vi "RS_RF_commands.vi"(1 "Value":dbl, 2 "Parameter":T1(ring)) -> (0 "Command":string)   [LabVIEW 2013]
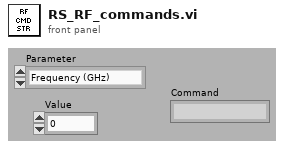
[diagram p1: front panel]
types:
  T1 = enum16{"Frequency (GHz)", "Power (dBm)", "Pulse period (us)", "Pulse width (us)", "Pulse delay (us)", "Pulse modulation?", "Output on?", "Pulse source", "Pulse mode", "Trigger mode", "Ex trigger input slope", "External impedance"}
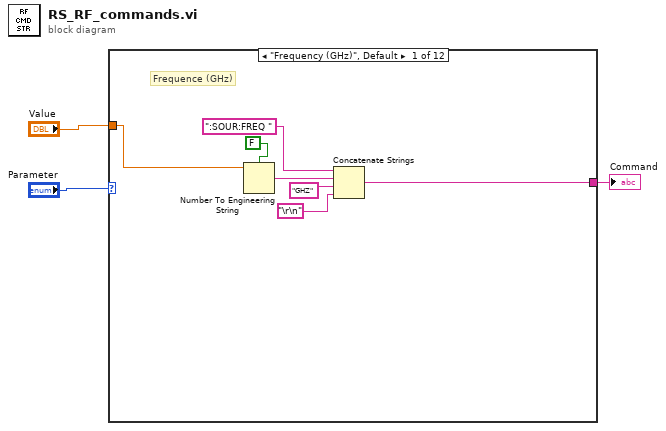
[diagram p0: block diagram]
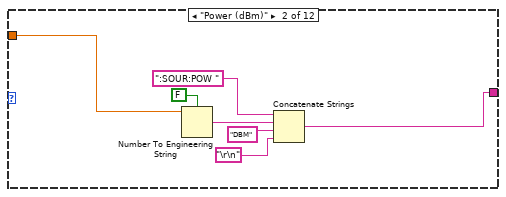
[diagram p2: hidden frame]
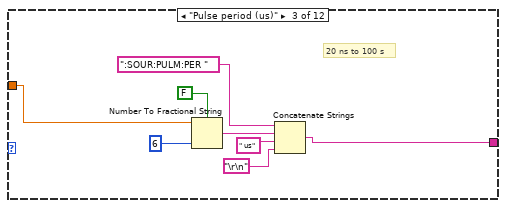
[diagram p3: hidden frame]
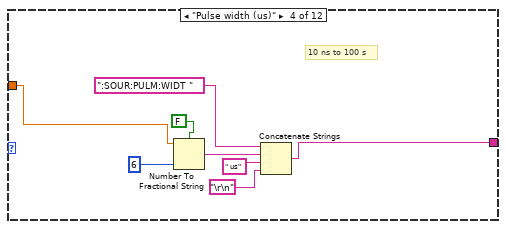
[diagram p4: hidden frame]
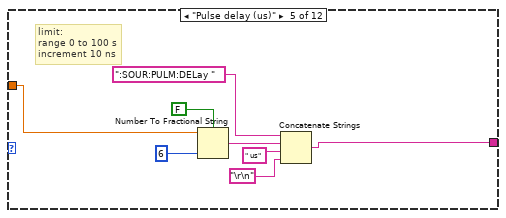
[diagram p5: hidden frame]
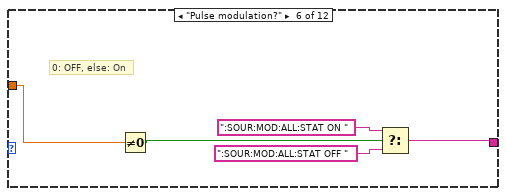
[diagram p6: hidden frame]
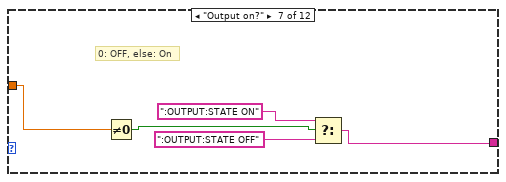
[diagram p7: hidden frame]
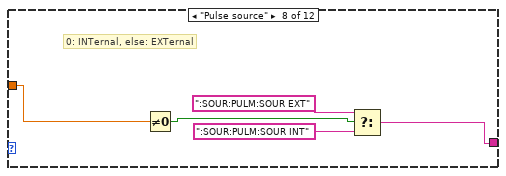
[diagram p8: hidden frame]
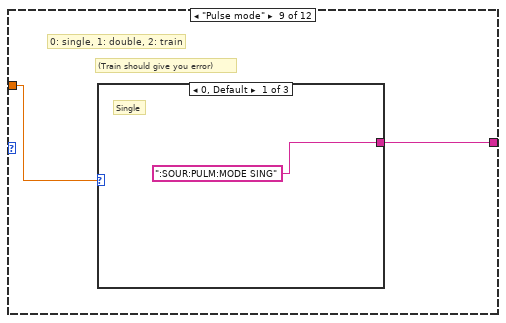
[diagram p9: hidden frame]
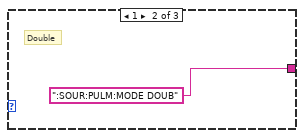
[diagram p10: hidden frame]
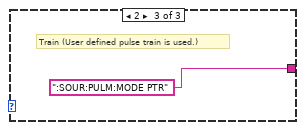
[diagram p11: hidden frame]
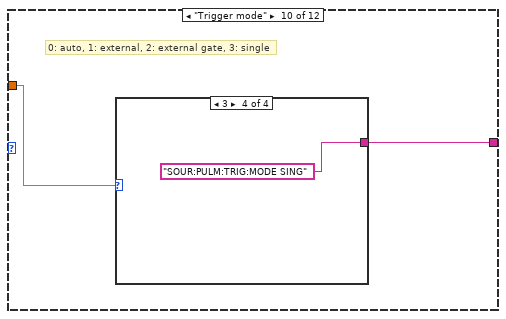
[diagram p12: hidden frame]
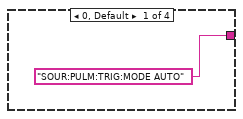
[diagram p13: hidden frame]
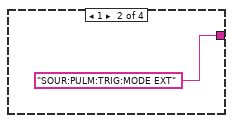
[diagram p14: hidden frame]
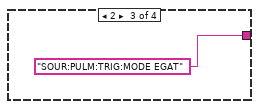
[diagram p15: hidden frame]
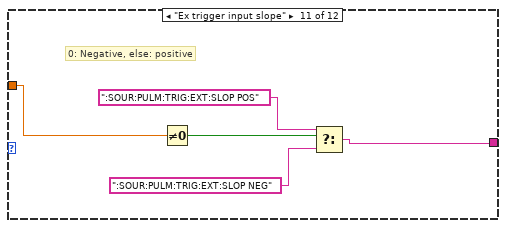
[diagram p16: hidden frame]
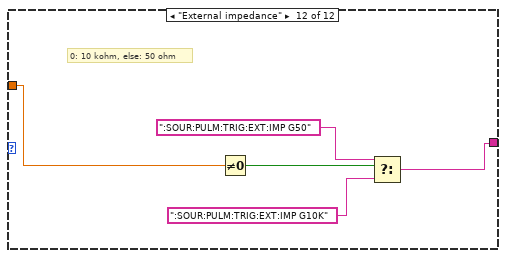
[diagram p17: hidden frame]
diagram:
  n1 = case shown="\"Frequency (GHz)\", Default" "Parameter" {
    tunnel: "Value" -> [w6 w14 w20 w27 w35 w44 w49 w53 w58 w63 w71 w74]
    tunnel: [w7 w13 w19 w28 w36 w42 w47 w52 w57 w62 w68 w73] -> w1
    frame "Frequency (GHz)", Default {
      # "Frequence (GHz)"
      n2 = Number To Engineering String(1:FALSE, 4:w6) -> (0:w8:string)  [unwired: 2 out]
      n3 = Concatenate Strings(":SOUR:FREQ " ("string"), w8, "GHZ" ("string"), "\r\n") -> (w7:string)
    }
    frame "Power (dBm)" {
      n4 = Number To Engineering String(1:FALSE, 4:w14) -> (0:w16:string)  [unwired: 2 out]
      n5 = Concatenate Strings(":SOUR:POW " ("string"), w16, "DBM" ("string"), "\r\n") -> (w13:string)
    }
    frame "Pulse period (us)" {
      # "20 ns to 100 s"
      n6 = Number To Fractional String(use system decimal point (T)=FALSE, number=w20, precision (6)=i16 6) -> (F-format string=w23:string)  [unwired: 1 in]
      n7 = Concatenate Strings(":SOUR:PULM:PER " ("string"), w23, " us" ("string"), "\r\n") -> (w19:string)
    }
    frame "Pulse width (us)" {
      # "10 ns to 100 s"
      n8 = Number To Fractional String(use system decimal point (T)=FALSE, number=w27, precision (6)=i16 6) -> (F-format string=w32:string)  [unwired: 1 in]
      n9 = Concatenate Strings(":SOUR:PULM:WIDT " ("string"), w32, " us" ("string"), "\r\n") -> (w28:string)
    }
    frame "Pulse delay (us)" {
      # "limit: \nrange 0 to 100 s \nincrement 10 ns"
      n10 = Number To Fractional String(use system decimal point (T)=FALSE, number=w35, precision (6)=i16 6) -> (F-format string=w39:string)  [unwired: 1 in]
      n11 = Concatenate Strings(":SOUR:PULM:DELay " ("string"), w39, " us" ("string"), "\r\n") -> (w36:string)
    }
    frame "Pulse modulation?" {
      # "0: OFF, else: On"
      n12 = Not Equal To 0?(x=w44) -> (x != 0?=w43:bool)
      n13 = Select(t=":SOUR:MOD:ALL:STAT ON " ("string"), s=w43, f=":SOUR:MOD:ALL:STAT OFF " ("string")) -> (s? t:f=w42:string)
    }
    frame "Output on?" {
      # "0: OFF, else: On"
      n14 = Not Equal To 0?(x=w49) -> (x != 0?=w48:bool)
      n15 = Select(t=":OUTPUT:STATE ON", s=w48, f=":OUTPUT:STATE OFF") -> (s? t:f=w47:string)
    }
    frame "Pulse source" {
      # "0: INTernal, else: EXTernal"
      n16 = Not Equal To 0?(x=w53) -> (x != 0?=w54:bool)
      n17 = Select(t=":SOUR:PULM:SOUR EXT", s=w54, f=":SOUR:PULM:SOUR INT") -> (s? t:f=w52:string)
    }
    frame "Pulse mode" {
      # "(Train should give you error)"
      # "0: single, 1: double, 2: train"
      n18 = case shown="0, Default" w58 {
        tunnel: [":SOUR:PULM:MODE SING" ":SOUR:PULM:MODE DOUB" ":SOUR:PULM:MODE PTR"] -> w57
        frame 0, Default {
          # "Single"
        }
        frame 1 {
          # "Double"
        }
        frame 2 {
          # "Train (User defined pulse train is used.)"
        }
      }
    }
    frame "Trigger mode" {
      # "0: auto, 1: external, 2: external gate, 3: single"
      n19 = case shown="3" w63 {
        tunnel: ["SOUR:PULM:TRIG:MODE AUTO" "SOUR:PULM:TRIG:MODE EXT" "SOUR:PULM:TRIG:MODE EGAT" "SOUR:PULM:TRIG:MODE SING"] -> w62
        frame 0, Default {
        }
        frame 1 {
        }
        frame 2 {
        }
        frame 3 {
        }
      }
    }
    frame "Ex trigger input slope" {
      # "0: Negative, else: positive"
      n20 = Not Equal To 0?(x=w71) -> (x != 0?=w72:bool)
      n21 = Select(t=":SOUR:PULM:TRIG:EXT:SLOP POS", s=w72, f=":SOUR:PULM:TRIG:EXT:SLOP NEG") -> (s? t:f=w68:string)
    }
    frame "External impedance" {
      # "0: 10 kohm, else: 50 ohm"
      n22 = Not Equal To 0?(x=w74) -> (x != 0?=w77:bool)
      n23 = Select(t=":SOUR:PULM:TRIG:EXT:IMP G50", s=w77, f=":SOUR:PULM:TRIG:EXT:IMP G10K") -> (s? t:f=w73:string)
    }
  }
  "Command" <- w1
